vi "set laser on.vi"(8 "error in (no error)":errorcluster, 11 "Cobolt in":refnum<class "Cobolt.lvclass">) -> (0 "error out":errorcluster, 3 "Cobolt out":refnum<class "Cobolt.lvclass">)   [LabVIEW 2012, in "Cobolt.lvclass"]
uses:
  Cobolt.lvclass
  CoboltLaserDrivers_Public_LV2012/CoboltLaser_Controls/ExpectedResponseType.ctl
  Cobolt.lvclass/Cobolt.ctl
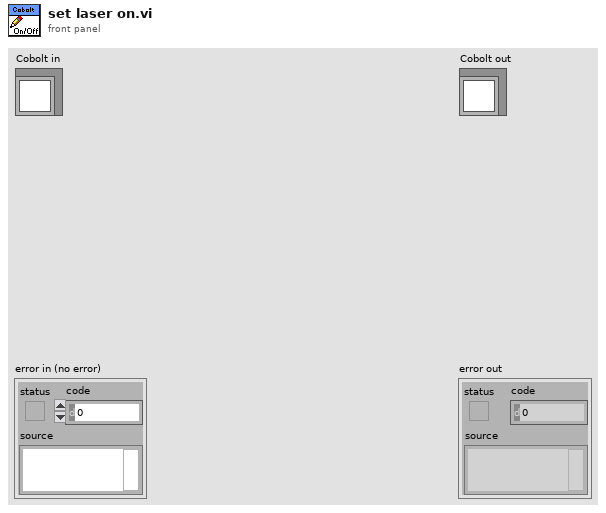
[diagram p1: front panel]
types:
  T1 = typedef "Cobolt.lvclass/ExpectedResponseType.ctl" = u16
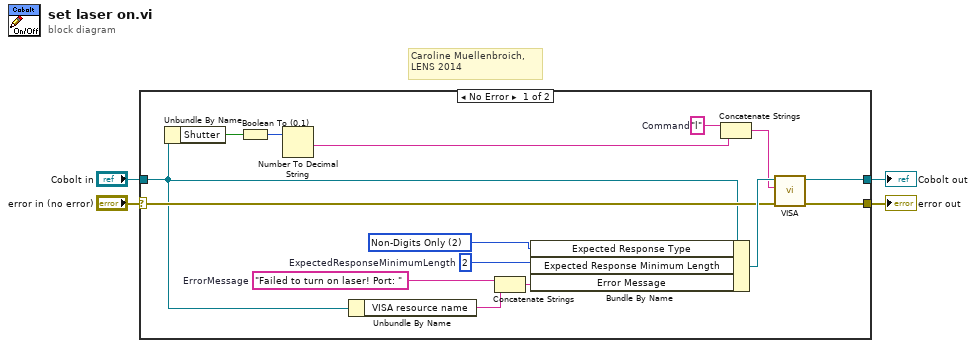
[diagram p0: block diagram]
diagram:
  # "Caroline Muellenbroich, \nLENS 2014"
  n1 = case shown="No Error" "error in (no error)" {
    selector: "error in (no error)" -> [w13 w21]
    tunnel: [w6 w21] -> w3
    tunnel: [w5 w20] -> w1
    tunnel: "Cobolt in" -> [w12 w20]
    frame No Error {
      w19 = T1 2 items=["Any", "Digits Only", "Non-Digits Only"] ("ExpectedResponseType")
      w15 = 2  # ExpectedResponseMinimumLength
      w17 = "Failed to turn on laser! Port: "  # ErrorMessage
      w8 = "l"  # Command
      n2 = Unbundle By Name(w12) -> ("Shutter"=w11:bool)
      n3 = Boolean To (0,1)(Boolean=w11) -> (0, 1=w10:i16)
      n4 = Number To Decimal String(number=w10) -> (decimal integer string=w7:string)  [unwired: 1 in]
      n5 = Unbundle By Name(w12) -> ("VISA resource name"=w16:string)
      n6 = Concatenate Strings(w17, w16) -> (w18:string)
      n7 = Bundle By Name(cluster=w12, "Expected Response Type"=w19, "Expected Response Minimum Length"=w15, "Error Message"=w18) -> (w14:refnum<class "Cobolt.lvclass">)
      n8 = Concatenate Strings(w8, w7) -> (w9:string)
      n9 = call-dynamic "VISA.vi"("error in (no error)"=w13, "string to write"=w9, "Cobolt in"=w14) -> ("error out"=w6:errorcluster, "Cobolt out"=w5:refnum<class "Cobolt.lvclass">)  [unwired: 6 in, 1 out]
    }
    frame Error {
    }
  }
  "error out" <- w3
  "Cobolt out" <- w1
